vi "Initialize_DMM.vi"(8 "error in (no error)":errorcluster, 10 "DMM_Initialize":T1, 11 "Keysight_34401A-DMM in":refnum<class "Keysight_34401A-DMM.lvclass">) -> (0 "error out":errorcluster, 3 "Keysight_34401A-DMM out":refnum<class "Keysight_34401A-DMM.lvclass">)   [LabVIEW 2020, in "Keysight_34401A-DMM.lvclass"]
uses:
  Keysight_34401A-DMM.lvclass
  C:/Program Files/National Instruments/LabVIEW 2020/vi.lib/MeasurementLink/MeasurementLink Instrument/ISession Factory/ISession Factory.lvclass
  DMM_Base/Typedef/DMM_Initialize.ctl
  <vilib>/MeasurementLink/MeasurementLink Session Management V1/Session Reservation/Initialize and Close Session Behavior.ctl
  Keysight_34401A-DMM.lvclass/Keysight_34401A-DMM.ctl
  8196af0f-1c90-4534-837c-d451b2e8b892.vi
  <vilib>/MeasurementLink/MeasurementLink Session Management V1/Session Reservation/Initialize Sessions with Retry.vi
  <vilib>/MeasurementLink/MeasurementLink Session Management V1/Session Reservation/Session Reservation.lvclass
  DMM_Base/DMM_Base.lvclass
panel:
  out "channel list":string
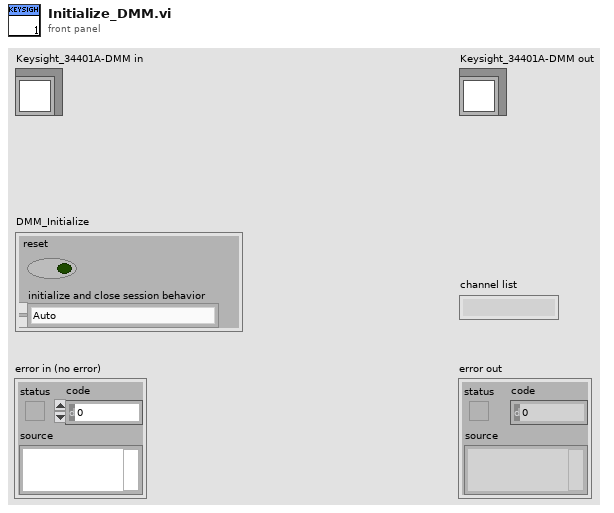
[diagram p1: front panel]
types:
  T1 = typedef "DMM_Base.lvclass/DMM_Initialize.ctl" = cluster{"initialize and close session behavior":T2, "reset":bool}
  T2 = typedef "MeasurementLink Session Management V1.lvlib/Session Reservation.lvclass/Initialize and Close Session Behavior.ctl" = enum16{"Auto", "Initialize and Close", "Attach and Detach", "Initialize and Detach", "Attach and Close"}
  T3 = cluster{"Baud Rate":u32, "Parity":u16, "Data Bits":u16}
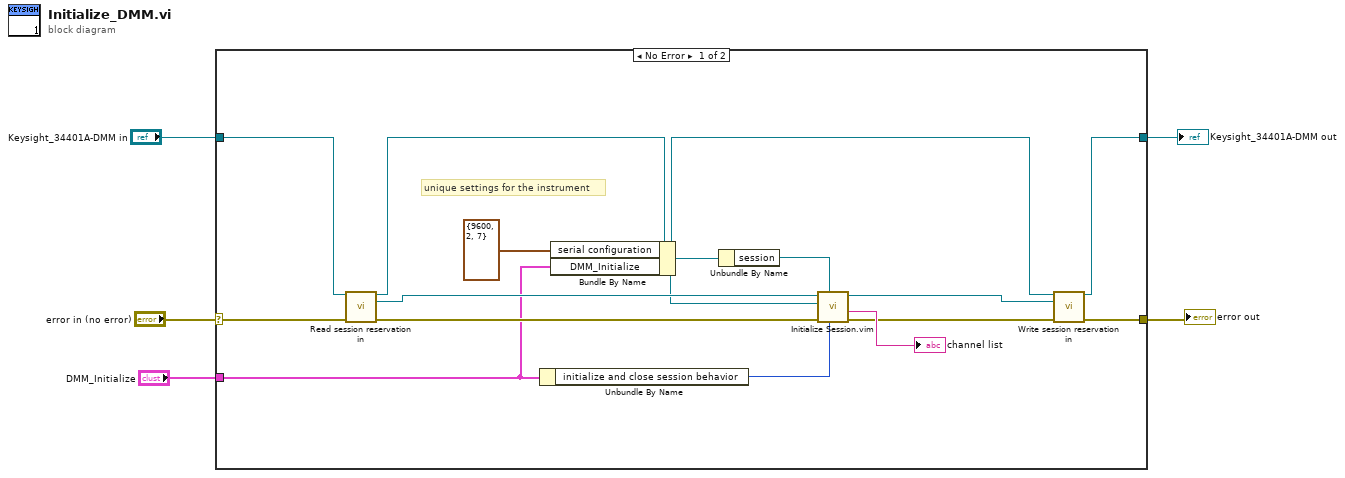
[diagram p0: block diagram]
diagram:
  n1 = case shown="No Error" "error in (no error)" {
    selector: "error in (no error)" -> [w10 w21]
    tunnel: [w9 w21] -> w4
    tunnel: [w8 w22] -> w3
    tunnel: "Keysight_34401A-DMM in" -> [w7 w22]
    tunnel: "DMM_Initialize" -> [w6 _]
    frame No Error {
      # "unique settings for the instrument"
      n2 = call-dynamic "Read session reservation in.vi"("AbstractDMM in"=w7, "error in (no error)"=w10) -> ("AbstractDMM out"=w20:refnum<class "Keysight_34401A-DMM.lvclass">, "MeasurementLink Session Management V1.lvlib:Session Reservation.lvclass"=w17:refnum<class "Session Reservation.lvclass">, "error out"=w18:errorcluster)  [unwired: 11 in]
      n3 = Unbundle By Name(w6) -> ("initialize and close session behavior"=w15:T2)
      n4 = Bundle By Name(cluster=w20, "serial configuration"=T3 {"Baud Rate"=9600, "Parity"=2, "Data Bits"=7}, "DMM_Initialize"=w6) -> (w12:refnum<class "Keysight_34401A-DMM.lvclass">)
      n5 = Unbundle By Name(w12) -> ("session"=w11:refnum<visa-resource-name>)
      n6 = call "Initialize Session.vim"("initialize and close session behavior"=w15, "session type"=w11, "error in"=w18, "session factory"=w12, "session reservation in"=w17) -> ("error out"=w14:errorcluster, "channel list"=→"channel list":string, "session reservation out"=w13:refnum<class "Session Reservation.lvclass">)  [unwired: 3 in, 1 out]
      n7 = call-dynamic "Write session reservation in.vi"("AbstractDMM in"=w12, "MeasurementLink Session Management V1.lvlib:Session Reservation.lvclass"=w13, "error in (no error)"=w14) -> ("AbstractDMM out"=w8:refnum<class "Keysight_34401A-DMM.lvclass">, "error out"=w9:errorcluster)  [unwired: 11 in]
    }
    frame Error {
    }
  }
  "error out" <- w4
  "Keysight_34401A-DMM out" <- w3
